vi "WPI_CameraManage Camera Settings.vi"(8 "Values In":T1, 9 "Value":i32, 10 "Operation":T2, 11 "Camera IP":string) -> (0 "Values":T1, 3 "Changed":bool)   [LabVIEW 2017]
doc: "Keep track of the currrent WPI camera settings. This is used to avoid redundant sets to the lower level camera drivers."
uses:
  <vilib>/Rock Robotics/WPI/Camera/WPI_CameraSettings Operations.ctl
  <vilib>/Rock Robotics/WPI/Camera/WPI_CameraSettings Control.ctl
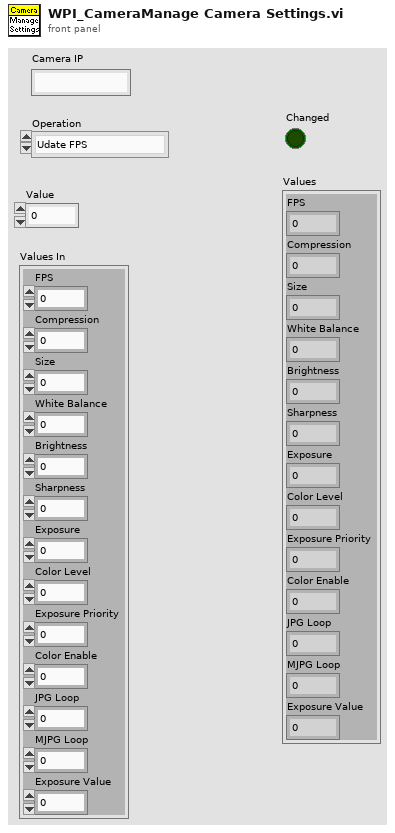
[diagram p1: front panel]
types:
  T1 = typedef "WPI_CameraSettings Control.ctl" = cluster{"FPS":i32, "Compression":i32, "Size":i32, "White Balance":i32, "Brightness":i32, "Sharpness":i32, "Exposure":i32, "Color Level":i32, "Exposure Priority":i32, "Color Enable":i32, "JPG Loop":i32, "MJPG Loop":i32, "Exposure Value":i32}
  T2 = typedef "WPI_CameraSettings Operations.ctl" = enum16{"Udate FPS", "Update Compression", "Update Size", "Update White Balance", "Update Brightness", "Update Sharpness", "Update Exposure", "Update Exposure Value", "Update Color Level", "Update Exp Priority", "Update Color Enable", "Update JPG", "Update MJPG", "Read and Clear", "Read", "Init"}
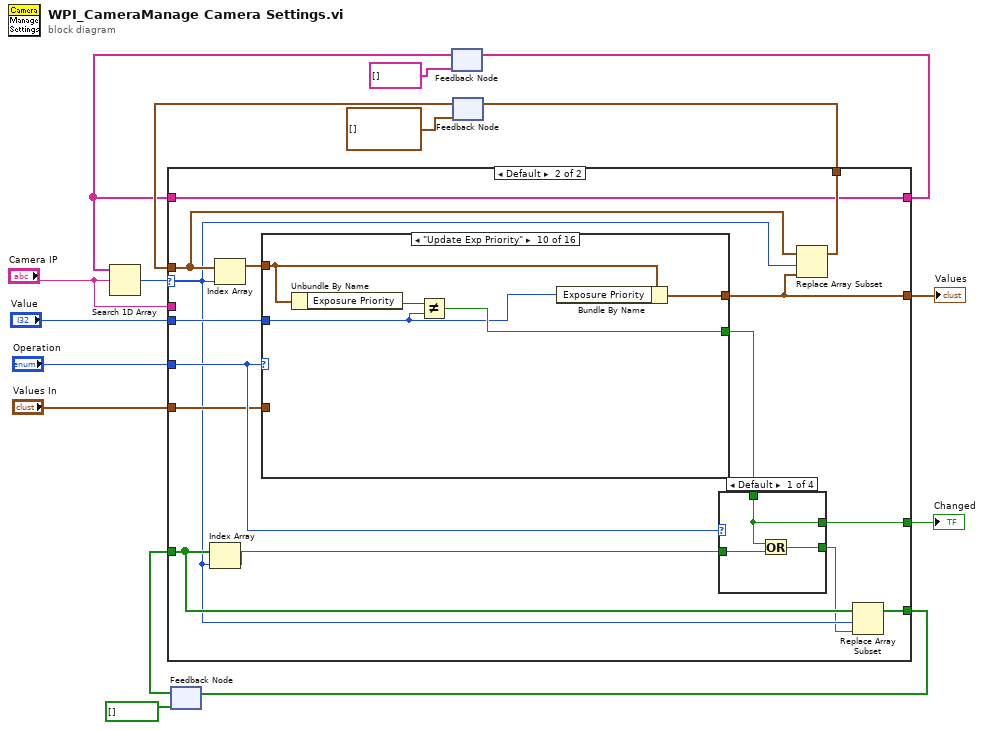
[diagram p0: block diagram]
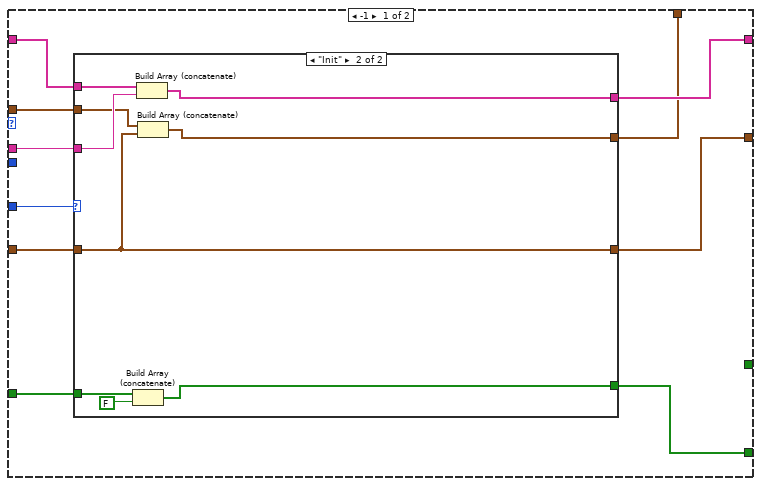
[diagram p2: hidden frame]
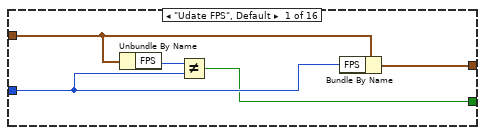
[diagram p7: hidden frame]
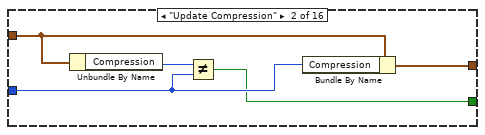
[diagram p8: hidden frame]
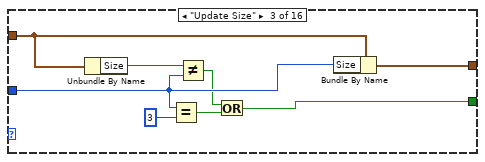
[diagram p9: hidden frame]
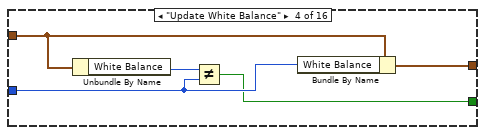
[diagram p10: hidden frame]
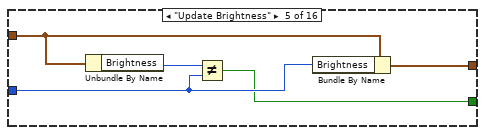
[diagram p11: hidden frame]
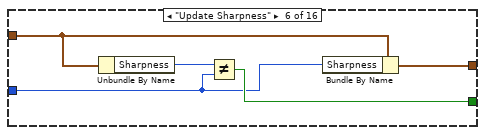
[diagram p12: hidden frame]
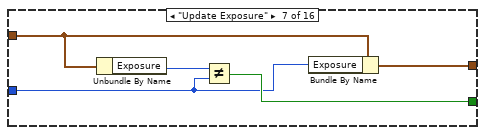
[diagram p13: hidden frame]
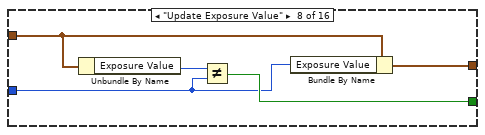
[diagram p14: hidden frame]
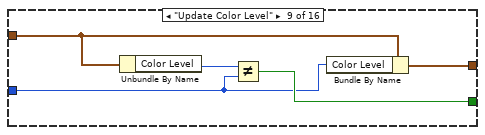
[diagram p15: hidden frame]
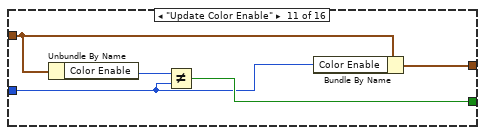
[diagram p16: hidden frame]
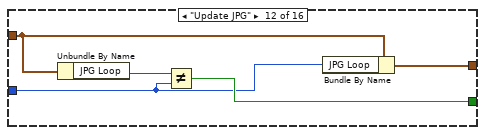
[diagram p17: hidden frame]
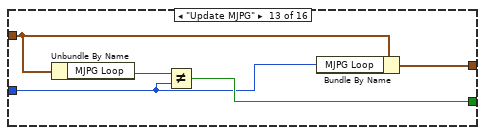
[diagram p18: hidden frame]
diagram:
  n1 = feedback #1(bool[] []) -> (w6:bool[])
  n2 = feedback #2(string[] []) -> (w2:string[])
  n3 = Search 1D Array(1D array=w2, element="Camera IP") -> (index of element=w7:i32)  [unwired: 1 in]
  n4 = feedback #3(T1[] []) -> (w9:T1[])
  n5 = case shown="Default" w7 {
    selector: w7 -> [_ w43]
    tunnel: "Value" -> [_ w54]
    tunnel: [w18 w48] -> w15
    tunnel: "Operation" -> [w26 w53]
    tunnel: [_ w51] -> w13
    tunnel: "Values In" -> [w19 w50]
    tunnel: w9 -> [w20 w46]
    tunnel: [w17 w47] -> w8
    tunnel: w6 -> [w22 w44]
    tunnel: [w21 w41] -> w4
    tunnel: [w25 w40] -> w3
    tunnel: w2 -> [w24 w40]
    tunnel: "Camera IP" -> [w23 _]
    frame -1 {
      n6 = case shown="\"Init\"" w26 {
        tunnel: [w30 w37] -> w25
        tunnel: w24 -> [w30 w39]
        tunnel: w23 -> [_ w38]
        tunnel: w22 -> [w29 w35]
        tunnel: [w29 w36] -> w21
        tunnel: w20 -> [w28 w33]
        tunnel: w19 -> [w27 w31]
        tunnel: [w28 w32] -> w18
        tunnel: [w27 w31] -> w17
        frame Default {
        }
        frame "Init" {
          n7 = Build Array (concatenate)(w35, FALSE) -> (w36:bool[])
          n8 = Build Array (concatenate)(w39, w38) -> (w37:string[])
          n9 = Build Array (concatenate)(w33, w31) -> (w32:T1[])
        }
      }
    }
    frame Default {
      n10 = Index Array(array=w44, index=w43) -> (element=w45:bool)
      n11 = Index Array(array=w46, index=w43) -> (element=w49:T1)
      n12 = case shown="\"Update Exp Priority\"" w53 {
        tunnel: w49 -> [w62 w68 w77 w80 w86 w91 w97 w99 w106 w111 w114 w119 w124 w128 w129 _]
        tunnel: w54 -> [w64 w67 w74 w79 w85 w89 w94 w100 w103 w108 w113 w118 w123 _ _ _]
        tunnel: [w63 w69 w75 w81 w87 w92 w96 w98 w107 w112 w115 w120 w125 w128 w129 w130] -> w47
        tunnel: [w60 w65 w70 w78 w83 w90 w95 w101 w104 w109 w116 w121 w126 _ _ _] -> w52
        tunnel: w50 -> [_ _ _ _ _ _ _ _ _ _ _ _ _ _ _ w130]
        frame "Udate FPS", Default {
          n13 = Unbundle By Name(w62) -> ("FPS"=w61:i32)
          n14 = Not Equal?(x=w61, y=w64) -> (x != y?=w60:bool)
          n15 = Bundle By Name(cluster=w62, "FPS"=w64) -> (w63:T1)
        }
        frame "Update Compression" {
          n16 = Unbundle By Name(w68) -> ("Compression"=w66:i32)
          n17 = Not Equal?(x=w66, y=w67) -> (x != y?=w65:bool)
          n18 = Bundle By Name(cluster=w68, "Compression"=w67) -> (w69:T1)
        }
        frame "Update Size" {
          n19 = Unbundle By Name(w77) -> ("Size"=w76:i32)
          n20 = Equal?(x=w74, y=3) -> (x = y?=w72:bool)
          n21 = Not Equal?(x=w76, y=w74) -> (x != y?=w71:bool)
          n22 = Or(x=w71, y=w72) -> (x .or. y?=w70:bool)
          n23 = Bundle By Name(cluster=w77, "Size"=w74) -> (w75:T1)
        }
        frame "Update White Balance" {
          n24 = Unbundle By Name(w80) -> ("White Balance"=w82:i32)
          n25 = Not Equal?(x=w82, y=w79) -> (x != y?=w78:bool)
          n26 = Bundle By Name(cluster=w80, "White Balance"=w79) -> (w81:T1)
        }
        frame "Update Brightness" {
          n27 = Unbundle By Name(w86) -> ("Brightness"=w84:i32)
          n28 = Not Equal?(x=w84, y=w85) -> (x != y?=w83:bool)
          n29 = Bundle By Name(cluster=w86, "Brightness"=w85) -> (w87:T1)
        }
        frame "Update Sharpness" {
          n30 = Unbundle By Name(w91) -> ("Sharpness"=w88:i32)
          n31 = Not Equal?(x=w88, y=w89) -> (x != y?=w90:bool)
          n32 = Bundle By Name(cluster=w91, "Sharpness"=w89) -> (w92:T1)
        }
        frame "Update Exposure" {
          n33 = Unbundle By Name(w97) -> ("Exposure"=w93:i32)
          n34 = Not Equal?(x=w93, y=w94) -> (x != y?=w95:bool)
          n35 = Bundle By Name(cluster=w97, "Exposure"=w94) -> (w96:T1)
        }
        frame "Update Exposure Value" {
          n36 = Unbundle By Name(w99) -> ("Exposure Value"=w102:i32)
          n37 = Not Equal?(x=w102, y=w100) -> (x != y?=w101:bool)
          n38 = Bundle By Name(cluster=w99, "Exposure Value"=w100) -> (w98:T1)
        }
        frame "Update Color Level" {
          n39 = Unbundle By Name(w106) -> ("Color Level"=w105:i32)
          n40 = Not Equal?(x=w105, y=w103) -> (x != y?=w104:bool)
          n41 = Bundle By Name(cluster=w106, "Color Level"=w103) -> (w107:T1)
        }
        frame "Update Exp Priority" {
          n42 = Unbundle By Name(w111) -> ("Exposure Priority"=w110:i32)
          n43 = Not Equal?(x=w110, y=w108) -> (x != y?=w109:bool)
          n44 = Bundle By Name(cluster=w111, "Exposure Priority"=w108) -> (w112:T1)
        }
        frame "Update Color Enable" {
          n45 = Unbundle By Name(w114) -> ("Color Enable"=w117:i32)
          n46 = Not Equal?(x=w117, y=w113) -> (x != y?=w116:bool)
          n47 = Bundle By Name(cluster=w114, "Color Enable"=w113) -> (w115:T1)
        }
        frame "Update JPG" {
          n48 = Unbundle By Name(w119) -> ("JPG Loop"=w122:i32)
          n49 = Not Equal?(x=w122, y=w118) -> (x != y?=w121:bool)
          n50 = Bundle By Name(cluster=w119, "JPG Loop"=w118) -> (w120:T1)
        }
        frame "Update MJPG" {
          n51 = Unbundle By Name(w124) -> ("MJPG Loop"=w127:i32)
          n52 = Not Equal?(x=w127, y=w123) -> (x != y?=w126:bool)
          n53 = Bundle By Name(cluster=w124, "MJPG Loop"=w123) -> (w125:T1)
        }
        frame "Read and Clear" {
        }
        frame "Read" {
        }
        frame "Init" {
        }
      }
      n54 = case shown="Default" w53 {
        tunnel: w45 -> [w57 w58 w59 _]
        tunnel: w52 -> [w55 _ _ _]
        tunnel: [w56 _ w59 _] -> w42
        tunnel: [w55 w58 w59 _] -> w51
        frame Default {
          n55 = Or(x=w55, y=w57) -> (x .or. y?=w56:bool)
        }
        frame "Read and Clear" {
        }
        frame "Read" {
        }
        frame "Init" {
        }
      }
      n56 = Replace Array Subset(array=w46, new element=w47, index=w43) -> (w48:T1[])
      n57 = Replace Array Subset(array=w44, new element=w42, index=w43) -> (w41:bool[])
    }
  }
  "Changed" <- w13
  "Values" <- w8
  n58 = feedback-in #1(w4) -> ()
  n59 = feedback-in #2(w3) -> ()
  n60 = feedback-in #3(w15) -> ()
